vi "Write Command Processor Status.vi"(8 "error in (no error)":errorcluster, 10 "Command Processor Status":T1, 11 "Command Processor in":refnum<class "Command Processor.lvclass">) -> (0 "error out":errorcluster, 3 "Command Processor out":refnum<class "Command Processor.lvclass">)   [LabVIEW 2014, in "Robot Actors.lvlib" / "Command Processor.lvlib" / "Command Processor.lvclass"]
uses:
  Command Processor.lvclass
  Command Processor Status.ctl
  Command/Command Class/Command Status.ctl
  Command/Command Class/Command States.ctl
  Command Processor States.ctl
  <vilib>/ActorFramework/Actor/Actor.lvclass/Actor.ctl
  Command Processor.lvclass/Command Processor.ctl
  System Actor/System Actor Messages/Updated Command Processor Status Msg/Updated Command Processor Status Msg.lvclass/Updated Command Processor Status Msg.ctl
  <vilib>/ActorFramework/Message Enqueuer/Message Enqueuer.lvclass/Message Enqueuer.ctl
  <vilib>/ActorFramework/Message Enqueuer/Enqueue.vi
  <vilib>/ActorFramework/Message Priority Queue/Priority Enqueue.vi
  System Actor/System Actor Messages/Updated Command Processor Status Msg/Updated Command Processor Status Msg.lvclass
  <vilib>/ActorFramework/Actor/Actor.lvclass
  Command/Command Class/Command.lvclass
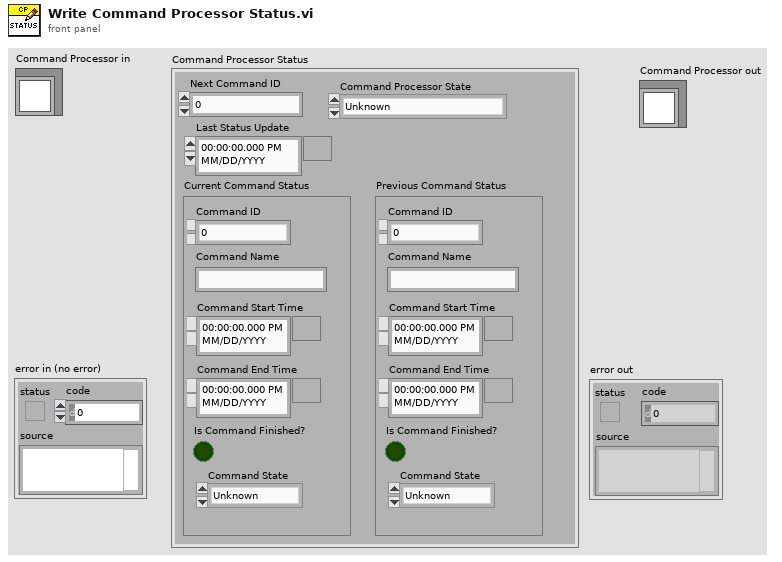
[diagram p1: front panel]
types:
  T1 = typedef "Robot Actors.lvlib/Command Processor.lvlib/Command Processor.lvclass/Command Processor Status.ctl" = cluster{"Next Command ID":dbl, "Current Command Status":T2, "Previous Command Status ":T2, "Command Processor State":T4, "Last Status Update":timestamp}
  T2 = typedef "Robot Actors.lvlib/Command.lvlib/Command.lvclass/Command Status.ctl" = cluster{"Command Name":string, "Command Start Time":timestamp, "Command End Time":timestamp, "Is Command Finished?":bool, "Command ID":dbl, "Command State":T3}
  T3 = typedef "Robot Actors.lvlib/Command.lvlib/Command.lvclass/Command States.ctl" = enum16{"Unknown", "Started", "Stopped", "Finished"}
  T4 = typedef "Robot Actors.lvlib/Command Processor.lvlib/Command Processor.lvclass/Command Processor States.ctl" = enum16{"Unknown", "No Command", "Running Command"}
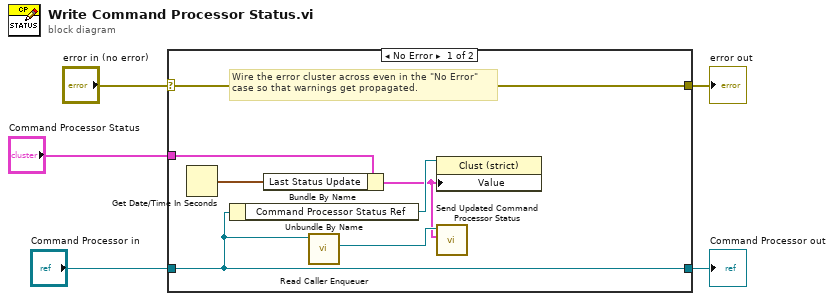
[diagram p0: block diagram]
diagram:
  n1 = case shown="No Error" "error in (no error)" {
    selector: "error in (no error)" -> [w12 w14]
    tunnel: [w12 w14] -> w4
    tunnel: [w10 w13] -> w2
    tunnel: "Command Processor in" -> [w10 w13]
    tunnel: "Command Processor Status" -> [w8 _]
    frame No Error {
      # "Wire the error cluster across even in the \"No Error\"\ncase so that warnings get propagated."
      n2 = Get Date/Time In Seconds() -> (seconds since 1Jan1904=w6:timestamp)
      n3 = Unbundle By Name(w10) -> ("Command Processor Status Ref"=w11:refnum<vi>)
      n4 = Bundle By Name(cluster=w8, "Last Status Update"=w6) -> (w7:T1)
      n5 = call <vilib>:"Read Caller Enqueuer.vi"("Actor"=w10) -> ("Caller Enqueuer"=w9:refnum<class "Message Enqueuer.lvclass">)  [unwired: 10 in]
      n6 = property class="Clust (strict)"(reference=w11, "Value"=w7) -> ()  [unwired: 1 in, 2 out]
      n7 = call "Send Updated Command Processor Status.vi"("Command Processor Status"=w7, "Message Enqueuer"=w9) -> ()  [unwired: 8 in, 2 out]
    }
    frame Error {
    }
  }
  "error out" <- w4
  "Command Processor out" <- w2
